vi "WSVCAP SHL Host TL SPI Write Read.vi"(0 "SPI Data Out":u8[][](array[numeric]) format="%.0x", 5 "Socket Mask":u16=1 format="%02x", 11 "error in":errorcluster, 13 "Log (T)":bool=TRUE) -> (4 "Read Data Out":u8[][](array[numeric]) format="%.0x", 15 "error out":errorcluster)   [LabVIEW 2012]
uses:
  Type Defs/WSVCAP SHL Function Enum.ctl
panel:
  out "Status":u8[](array[numeric])
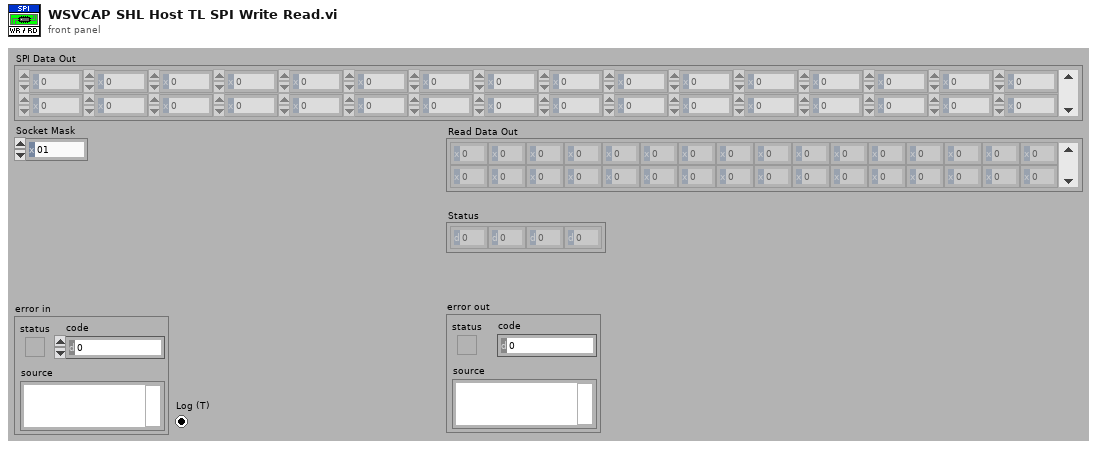
[diagram p1: front panel]
types:
  T1 = typedef "WSVCAP SHL Function Enum.ctl" = enum16{"Initialize", "Configure I2C", "Configure SPI", "Configure RFFE", "Write I2C", "Read I2C", "Write/Read SPI", "Start SPI Cycle", "Stop SPI Cycle", "Write RFFE", "Read RFFE", "Start RFFE Cycle", "Stop RFFE Cycle", "Get Status", "Close"}
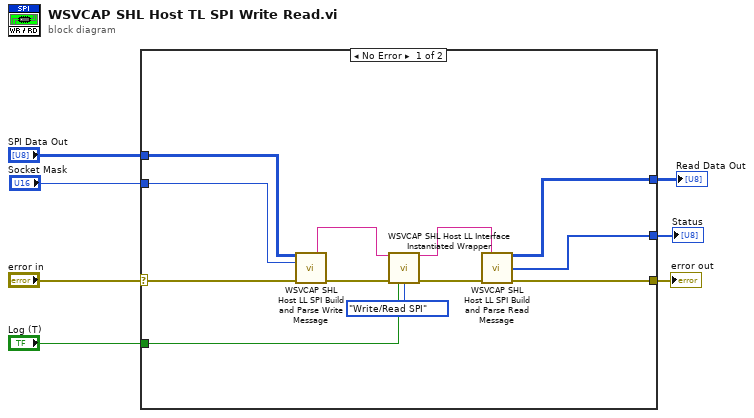
[diagram p0: block diagram]
diagram:
  n1 = case shown="No Error" "error in" {
    selector: "error in" -> [w14 w20]
    tunnel: [w13 w20] -> w7
    tunnel: "SPI Data Out" -> [w12 _]
    tunnel: "Socket Mask" -> [w8 _]
    tunnel: [w11 _] -> w3
    tunnel: [w10 _] -> w2
    tunnel: "Log (T)" -> [w9 _]
    frame No Error {
      n2 = call "WSVCAP SHL Host LL SPI Build and Parse Write Message.vi"("Write Data In [DUT Ordered]"=w12, "Socket Mask [U16] In"=w8, "error in"=w14) -> ("Message Out"=w16:string, "error out"=w18:errorcluster)  [unwired: 7 in, 4 out]
      n3 = call "WSVCAP SHL Host LL Interface Instantiated Wrapper.vi"("Message In"=w16, "error in"=w18, "Log (T)"=w9, "Function"=WSVCAP_SHL_Function_Enum."Write/Read SPI") -> ("Message Out"=w15:string, "error out"=w17:errorcluster)  [unwired: 9 in, 1 out]
      n4 = call "WSVCAP SHL Host LL SPI Build and Parse Read Message.vi"("Message In"=w15, "error in"=w17) -> ("Write Data Out"=w11:u8[][], "Status"=w10:u8[], "error out"=w13:errorcluster)  [unwired: 10 in, 1 out]
    }
    frame Error {
    }
  }
  "error out" <- w7
  "Read Data Out" <- w3
  "Status" <- w2
